vi "GetShiftTime.vi"(8 "error in (no error)":errorcluster, 11 "Time":timestamp) -> (0 "error out":errorcluster, 1 "Shift Elapsed Time [s]":dbl, 2 "Shift Start Time":timestamp, 3 "Shift End Time":timestamp)   [LabVIEW 2016]
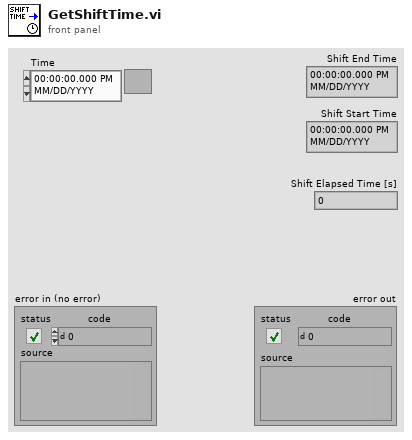
[diagram p1: front panel]
types:
  T1 = typedef "LVDateTimeRec.ctl" = cluster{"fractional second":dbl, "second":i32, "minute":i32, "hour":i32, "day of month":i32, "month":i32, "year":i32, "day of week":i32, "day of year":i32, "DST":i32}
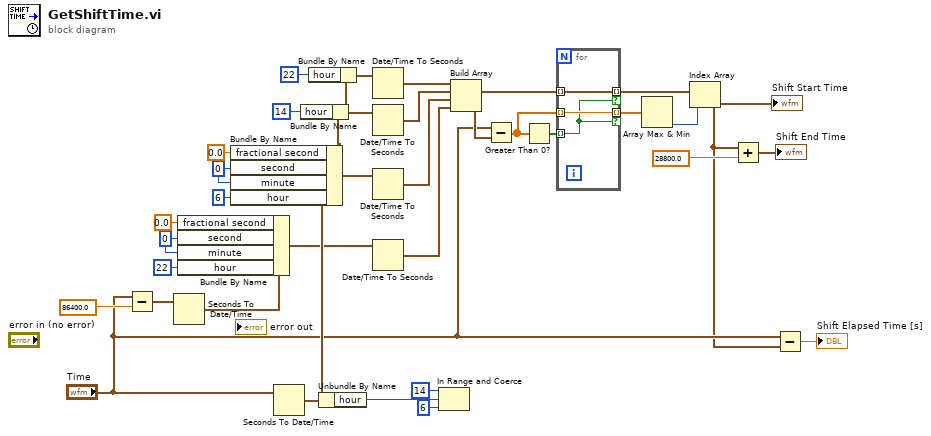
[diagram p0: block diagram]
diagram:
  w11 = 0 ("second")
  w30 = 0 ("second")
  n1 = Subtract(x="Time", y=86400.0 ("fractional second")) -> (x-y=w13:timestamp)
  n2 = Seconds To Date/Time(time stamp (now)=w13) -> (date time rec=w9:T1)  [unwired: 1 in]
  n3 = Bundle By Name(cluster=w9, "fractional second"=0.0, "second"=w11, "minute"=w11, "hour"=22) -> (w8:T1)
  n4 = Seconds To Date/Time(time stamp (now)="Time") -> (date time rec=w29:T1)  [unwired: 1 in]
  n5 = Bundle By Name(cluster=w29, "fractional second"=0.0, "second"=w30, "minute"=w30, "hour"=6) -> (w25:T1)
  n6 = Bundle By Name(cluster=w25, "hour"=14) -> (w24:T1)
  n7 = Bundle By Name(cluster=w24, "hour"=22) -> (w23:T1)
  n8 = Unbundle By Name(w29) -> ("hour"=w33:i32)
  n9 = Date/Time To Seconds(2:w23) -> (0:w22:timestamp)  [unwired: 1 in]
  n10 = Date/Time To Seconds(2:w24) -> (0:w21:timestamp)  [unwired: 1 in]
  n11 = Date/Time To Seconds(2:w25) -> (0:w20:timestamp)  [unwired: 1 in]
  n12 = Date/Time To Seconds(2:w8) -> (0:w7:timestamp)  [unwired: 1 in]
  n13 = In Range and Coerce(upper limit=14, x=w33, lower limit=6) -> ()  [unwired: 2 out]
  n14 = Build Array(w22, w21, w20, w7) -> (w19:timestamp[])
  n15 = Subtract(x="Time", y=w19) -> (x-y=w4:dbl[])
  n16 = Greater Than 0?(x=w4) -> (x > 0?=w18:bool[])
  n17 = for {
    tunnel: w19 -> [w37] mode=indexing
    tunnel: [w37] -> w17 mode=indexing if=w35
    tunnel: w18 -> [w35] mode=indexing
    tunnel: [w36] -> w16 mode=indexing if=w35
    tunnel: w4 -> [w36] mode=indexing
  }
  n18 = Array Max & Min(array=w16) -> (min index (indices)=w15:i32)  [unwired: 3 out]
  n19 = Index Array(array=w17, index=w15) -> (element=w2:timestamp)
  "Shift Start Time" <- w2
  n20 = Add(x=w2, y=28800.0 ("fractional second")) -> (x+y=→"Shift End Time":timestamp)
  n21 = Subtract(x="Time", y=w2) -> (x-y=→"Shift Elapsed Time [s]":dbl)
